vi "Open.vi"(8 "error in":errorcluster, 9 "parameters":variant, 10 "file path":path, 11 "CEF_Repository in":refnum<class "CEF_Repository.lvclass">) -> (0 "error out":errorcluster, 2 "invalid?":bool, 3 "CEF_Repository out":refnum<class "CEF_Repository.lvclass">)   [LabVIEW 2025, in "CEF.lvlib" / "CEF_Repository.lvclass"]
doc: "Loads the saved information of the repo. It could load multiple files at the same time. An option to add file versioning could be included in the files, and the code to manage changes would be in this VI.Copyright 2017 National Instruments Corporation\n\nLicensed under the Apache License, Version 2.0 (the \"License\"); you may not use this file except in compliance with the License. You may obtain a copy of the License at http://www.apache.org/licenses/LICENSE-2.0\nUnless required by applicable law or agreed to in writing, software distributed under the License is distributed on an \"AS IS\" BASIS, WITHOUT WARRANTIES OR CONDITIONS OF ANY KIND, either express or implied. See the License for the specific language governing permissions and limitations under the License."
uses:
  CEF_Repository.lvclass
  CEF.lvlib
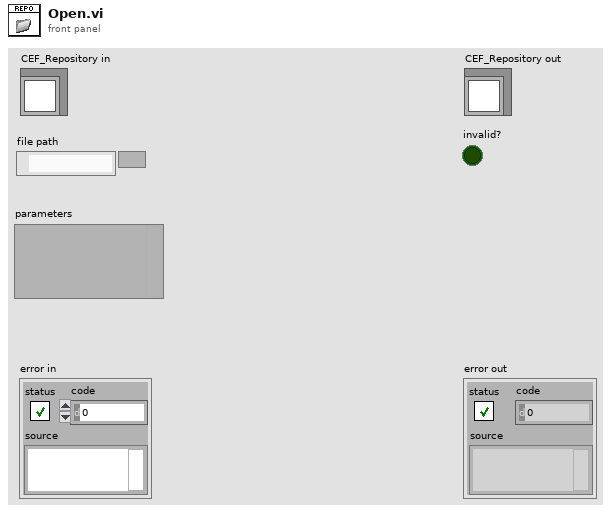
[diagram p1: front panel]
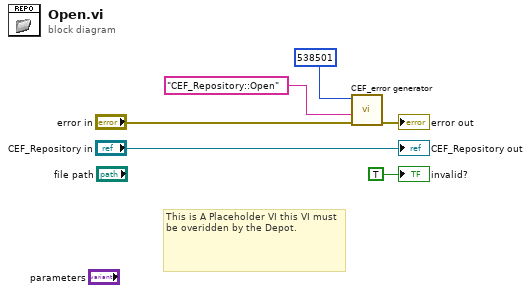
[diagram p0: block diagram]
diagram:
  # "This is A Placeholder VI this VI must be overidden by the Depot."
  n1 = call "CEF_error generator.vi"("error in"="error in", "source"="CEF_Repository::Open", "error code (0)"=538501) -> ("error out"=→"error out":errorcluster)  [unwired: 6 in]
  "CEF_Repository out" <- "CEF_Repository in"
  "invalid?" <- TRUE
